vi "Perspective_Globals.vi"() -> ()   [LabVIEW 2022 SP3]
panel:
  out "Outlines?":bool
  in  "correction":dbl
  in  "gap offset %":dbl=0.2
  in  "Rainbow":u32[](array[colorbox])=[7602431, 8126719, 7864574, 7536895, 7274750, 6947071, 6684926, 6357247, 6095102, 5767423, 5505278, 5177599, 4915454, 4587775, 4325630, 3997951, 3735806, 3408127, 3145982, 2818303, 2556158, 2228479, 1966334, 1638655, 1376510, 1048831, 786686, 459007, 196862, 767, 1790, 3071, 4094, 5375, 6398, 7679, 8702, 9983, 11006, 12287, 13310, 14591, 15614, 16895, 17918, 19199, 20222, 21503, 22526, 23807, 24830, 26111, 27134, 28415, 29438, 30719, 31486, 33023, 33790, 35327, 36094, 37631, 38398, 39935, 40702, 42239, 43006, 44543, 45310, 46847, 47614, 49151, 49918, 51455, 52222, 53759, 54526, 56063, 56830, 58367, 59134, 60671, 61694, 62975, 63998, 65279, 65274, 65527, 65265, 65518, 65256, 65509, 65247, 65500, 65238, 65491, 65229, 65482, 65220, 65473, 65211, 65464, 65202, 65455, 65193, 65446, 65184, 65437, 65175, 65428, 65166, 65419, 65157, 65410, 65149, 65401, 65140, 65392, 65131, 65383, 65122, 65374, 65113, 65365, 65104, 65356, 65095, 65347, 65086, 65338, 65077, 65329, 65068, 65320, 65059, 65311, 65050, 65302, 65041, 65293, 65032, 65284, 130560, 392960, 720384, 982784, 1310208, 1572608, 1900032, 2162432, 2489856, 2752256, 3079680, 3342080, 3669504, 3931904, 4259328, 4521728, 4849152, 5111552, 5438976, 5701376, 6028800, 6291200, 6618624, 6881024, 7208448, 7470848, 7798272, 8126208, 8322560, 8716032, 8912384, 9305856, 9502208, 9895680, 10092032, 10485504, 10681856, 11075328, 11271680, 11665152, 11861504, 12254976, 12451328, 12844800, 13041152, 13434624, 13630976, 14024448, 14220800, 14614272, 14810624, 15204096, 15400448, 15793920, 15990272, 16383744, 16580096, 16776192, 16709376, 16773888, 16707072, 16771584, 16704768, 16769280, 16702464, 16766976, 16700160, 16764672, 16697856, 16762368, 16695552, 16760064, 16693248, 16757760, 16690944, 16755456, 16688640, 16753152, 16686336, 16750848, 16684032, 16748544, 16681728, 16746240, 16679680, 16743936, 16677376, 16741632, 16675072, 16739328, 16672768, 16737024, 16670464, 16734720, 16668160, 16732416, 16665856, 16730112, 16663552, 16727808, 16661248, 16725504, 16658944, 16723200, 16656640, 16720896, 16654336, 16718592, 16652032, 16716288, 16649728, 16713984, 16712960, 15663104]
  in  "X,Y pixels":dbl=5.0
  in  "Z Height":i32=40
  in  "vanishing points":cluster{"x":dbl, "y":dbl}[](array[cluster])=[{"x"=-400.0, "y"=200.0}, {"x"=400.0, "y"=200.0}]
  in  "origin":cluster{"x":dbl, "y":dbl}={"x"=300.0, "y"=200.0}
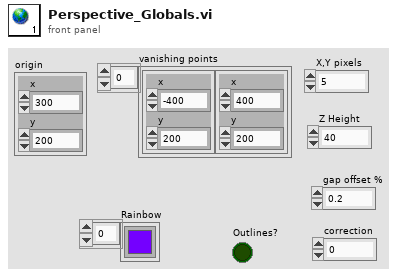
[diagram p1: front panel]
diagram:
